vi "Analyze.vi"(8 "error in (no error)":errorcluster, 10 "Image in":T1, 11 "Analyze Distanz in":refnum<class "Analyze BeamDeviation.lvclass">) -> (0 "error out":errorcluster, 1 "Result":refnum<class "Analyze Results Base.lvclass">, 2 "Image out":T1, 3 "Analyze Distanz out":refnum<class "Analyze BeamDeviation.lvclass">)   [LabVIEW 2020, in "Analyze.lvlib" / "Analyze BeamDeviation.lvclass"]
uses:
  Analyze BeamDeviation.lvclass
  C:/Users/AlexK/work/LabVIEW Programme/POLARIS-AS-3-Cams/Submodules/HIJ Vision/Analyze/Analyze Classes/Analyze BaseClass/Analyze BaseClass/Analyze BaseClass.lvclass
  <vilib>/vision/Image Controls.llb/IMAQ Image.ctl
  Results and Overlays/Results Base/Analyze Results Base.lvclass
  Results and Overlays/Results Beam Deviation/Analyze Results Beam Deviation.lvclass
  C:/Users/AlexK/work/LabVIEW Programme/POLARIS-AS-3-Cams/Submodules/HIJ Vision/Analyze/Results and Overlays/Results Base/Analyze Results Base.lvclass
  Analyze Parameter/Analyze Parameter Target Point/Target Point.lvclass
  C:/Users/AlexK/work/LabVIEW Programme/POLARIS-AS-3-Cams/Submodules/HIJ Vision/Analyze/Analyze Parameter/Analyze Parameter Base/Analyze Parameter Base.lvclass
  Analyze Parameter/Analyze Parameter Target Point/Target Point.lvclass/Target Point.ctl
  Results and Overlays/Results Beam Deviation/Analyze Results Beam Deviation.lvclass/Analyze Results Beam Deviation.ctl
  Results and Overlays/Results Beam Deviation/Write Delta.vi
  Analyze BaseClass/Analyze BaseClass/Analyze BaseClass.lvclass
  Analyze BeamDeviation.lvclass/Analyze BeamDeviation.ctl
  <vilib>/vision/NI_Vision_Development_Module.lvlib
  C:/Program Files (x86)/National Instruments/LabVIEW 2020/vi.lib/ActorFramework/Actor/Actor.lvclass
  C:/Users/AlexK/work/LabVIEW Programme/POLARIS-AS-3-Cams/Submodules/HIJ Vision/Analyze/Analyze Classes/Analyze Diviation/Analyze BeamDeviation.lvclass
  C:/Users/AlexK/work/LabVIEW Programme/POLARIS-AS-3-Cams/Submodules/HIJ Vision/Analyze/Results and Overlays/Results Beam Deviation/Analyze Results Beam Deviation.lvclass
  C:/Users/AlexK/work/LabVIEW Programme/POLARIS-AS-3-Cams/Submodules/HIJ Vision/Analyze/Analyze Parameter/Analyze Parameter Target Point/Target Point.lvclass
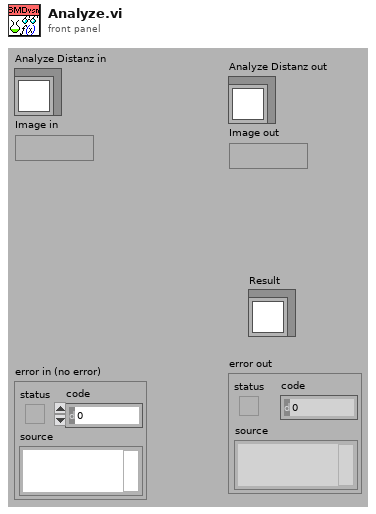
[diagram p1: front panel]
types:
  T1 = typedef "IMAQ Image.ctl" = refnum<image>
  T2 = typedef "ROI Descriptor" = cluster{"Global Rectangle":i32[], "Contours":cluster{"ID":enum32{"External", "Internal"}, "Type":u32, "Coordinates":i32[]}[]}
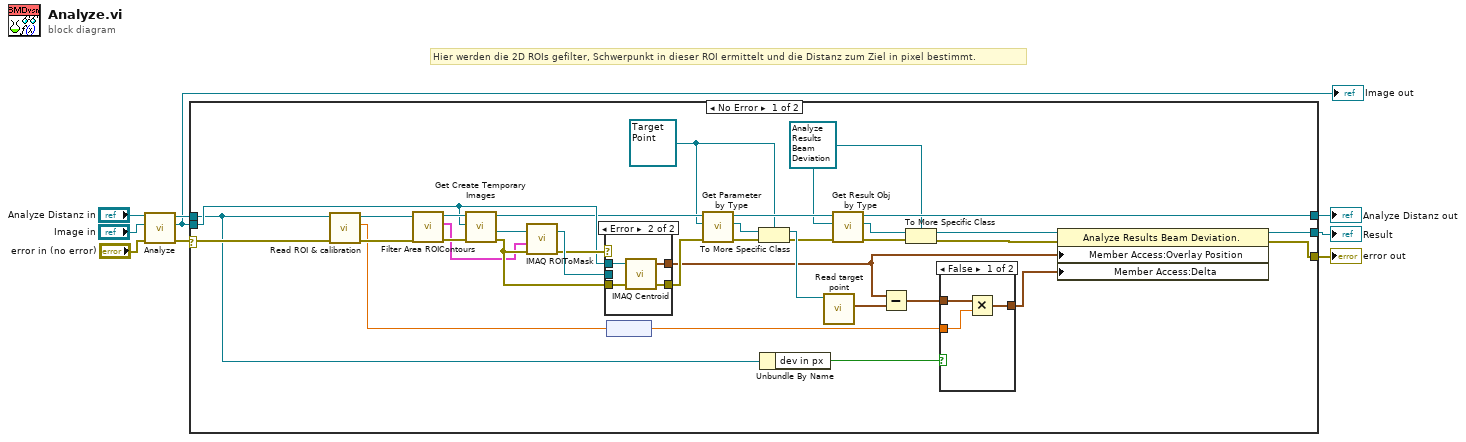
[diagram p0: block diagram]
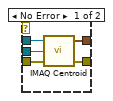
[diagram p3: hidden frame]
diagram:
  # "Hier werden die 2D ROIs gefilter, Schwerpunkt in dieser ROI ermittelt und die Distanz zum Ziel in pixel bestimmt."
  n1 = call-parent "Analyze.vi"("error in (no error)"="error in (no error)", "Image in"="Image in", "Analyze BaseClass in"="Analyze Distanz in") -> ("error out"=w1:errorcluster, "Image out"=w5:T1, "Analyze BaseClass out"=w7:refnum<class "Analyze BeamDeviation.lvclass">)  [unwired: 5 in, 1 out]
  "Image out" <- w5
  n2 = case shown="No Error" w1 {
    selector: w1 -> [w17 w59]
    tunnel: w7 -> [w11 w58]
    tunnel: w5 -> [w37 _]
    tunnel: [w34 _] -> w4
    tunnel: [w33 w59] -> w3
    tunnel: [w25 w58] -> w2
    frame No Error {
      w29 = refnum<class "Target Point.lvclass"> refnum ("Target Point.lvclass")
      w24 = refnum<class "Analyze Results Beam Deviation.lvclass"> refnum ("Analyze Results Beam Deviation.lvclass")
      n3 = call-dynamic "Read ROI & calibration.vi"("error in (no error)"=w17, "Analyze BaseClass in"=w11) -> ("error out"=w16:errorcluster, "calibration mm/px"=w14:dbl[unit], "Analyze BaseClass out"=w18:refnum<class "Analyze BeamDeviation.lvclass">)  [unwired: 6 in, 1 out]
      n4 = call-dynamic "Filter Area ROIContours.vi"("error in (no error)"=w16, "Analyze BaseClass in"=w18) -> ("error out"=w43:errorcluster, "ROI of Area type"=w38:T2, "Analyze BaseClass out"=w44:refnum<class "Analyze BeamDeviation.lvclass">)  [unwired: 7 in]
      n5 = call-dynamic "Get Create Temporary Images.vi"("error in (no error)"=w43, "Image in"=w37, "Analyze BaseClass in"=w44) -> ("error out"=w40:errorcluster, "image mask"=w42:T1, "Analyze BaseClass out"=w35:refnum<class "Analyze BeamDeviation.lvclass">)  [unwired: 4 in, 2 out]
      n6 = call "IMAQ ROIToMask"("error in (no error)"=w40, "ROI Descriptor"=w38, "Image"=w42) -> ("error out"=w39:errorcluster, "Image Out"=w41:T1)  [unwired: 3 in, 1 out]
      n7 = case shown="Error" w39 {
        tunnel: w37 -> [w53 w57]
        tunnel: w41 -> [w52 _]
        tunnel: [w51 w56] -> w27
        tunnel: [w50 w55] -> w12
        tunnel: w40 -> [w49 w54]
        frame No Error {
          n8 = call "IMAQ Centroid"("error in (no error)"=w49, "Image Mask"=w52, "Image"=w53) -> ("error out"=w51:errorcluster, "Centroid"=w50:cluster{"X Centroid":sgl, "Y Centroid":sgl})  [unwired: 1 in]
        }
        frame Error {
          n9 = call "IMAQ Centroid"("error in (no error)"=w54, "Image"=w57) -> ("error out"=w56:errorcluster, "Centroid"=w55:cluster{"X Centroid":sgl, "Y Centroid":sgl})  [unwired: 2 in]
        }
      }
      n10 = node(w14) -> (w13:dbl)
      n11 = call "Get Parameter by Type.vi"("error in (no error)"=w27, "Parameter Type"=w29, "Analyze BaseClass in"=w35) -> ("error out"=w26:errorcluster, "Parameter"=w28:refnum<class "Analyze Parameter Base.lvclass">, "Analyze BaseClass out"=w30:refnum<class "Analyze BeamDeviation.lvclass">)  [unwired: 5 in, 1 out]
      n12 = To More Specific Class(target class=w29, reference=w28, error in=w26) -> (specific class reference=w31:refnum<class "Target Point.lvclass">, error out=w20:errorcluster)
      n13 = Unbundle By Name(w11) -> ("dev in px"=w10:bool)
      n14 = call "Read target point.vi"("Target Point in"=w31) -> ("target point"=w36:cluster{"x":i16, "y":i16})  [unwired: 8 in, 2 out]
      n15 = call "Get Result Obj by Type.vi"("error in (no error)"=w20, "Parameter Type"=w24, "Analyze BaseClass in"=w30) -> ("error out"=w21:errorcluster, "Parameter"=w23:refnum<class "Analyze Results Base.lvclass">, "Analyze BaseClass out"=w25:refnum<class "Analyze BeamDeviation.lvclass">)  [unwired: 5 in, 1 out]
      n16 = Subtract(x=w12, y=w36) -> (x-y=w32:cluster{sgl, sgl})
      n17 = To More Specific Class(target class=w24, reference=w23, error in=w21) -> (specific class reference=w22:refnum<class "Analyze Results Beam Deviation.lvclass">, error out=w19:errorcluster)
      n18 = case shown="False" w10 {
        tunnel: w32 -> [w47 w48]
        tunnel: [w46 w48] -> w15
        tunnel: w13 -> [w45 _]
        frame False {
          n19 = Multiply(x=w47, y=w45) -> (x*y=w46:cluster{dbl, dbl})
        }
        frame True {
        }
      }
      n20 = property class="Analyze Results Beam Deviation."(reference=w22, error in=w19, "Member Access:Overlay Position"=w12, "Member Access:Delta"=w15) -> (reference out=w34:refnum<class "Analyze Results Beam Deviation.lvclass">, error out=w33:errorcluster)
    }
    frame Error {
    }
  }
  "error out" <- w3
  "Analyze Distanz out" <- w2
  "Result" <- w4
